vi "Test_Get Meta Details.vi"() -> ()   [LabVIEW 2020, in "Measurement Client Wrapper.lvclass"]
uses:
  Measurement Client Wrapper.lvclass
panel:
  out "Measurement Client Wrapper out":refnum<class "Measurement Client Wrapper.lvclass">
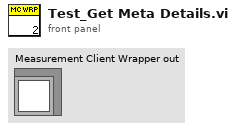
[diagram p1: front panel]
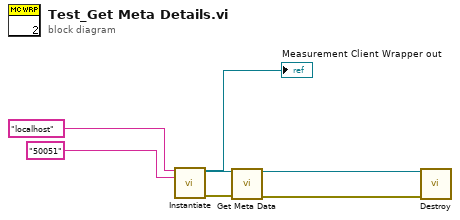
[diagram p0: block diagram]
diagram:
  n1 = call "Instantiate.vi"("location"="localhost", "insecurePort"="50051") -> ("Measurement Client Wrapper out"=w3:refnum<class "Measurement Client Wrapper.lvclass">, "error out"=w4:errorcluster)  [unwired: 12 in]
  "Measurement Client Wrapper out" <- w3
  n2 = call "Get Meta Data.vi"("Measurement Client Wrapper in"=w3, "error in"=w4) -> ("Measurement Client Wrapper out"=w2:refnum<class "Measurement Client Wrapper.lvclass">, "error out"=w1:errorcluster)  [unwired: 12 in]
  n3 = call "Destroy.vi"("Measurement Client Wrapper in"=w2, "error in"=w1) -> ()  [unwired: 12 in, 2 out]
